vi "Convert API String Arguments to Data(variant).vi"(7 "Type":variant, 9 "error in (no error)":errorcluster, 10 "Strict Label Check?(T)":bool=TRUE, 11 "String":string) -> (1 "error":errorcluster, 3 "Data":variant)   [LabVIEW 2017, in "API String Arguments Support.lvlib"]
uses:
  API String Arguments Support.lvlib
  <vilib>/Utility/Data Type/Type Definitions/Data Type.ctl
  <vilib>/Utility/Data Type/Type Definitions/Tag Type.ctl
  <vilib>/Utility/Data Type/Type Definitions/Refnum Type.ctl
  <userlib>/_NEVSTOP/Communicable State Machine(CSM)/AdvanceAPI/CSM - Keywords.vi
  <vilib>/Utility/Data Type/NI_Data Type.lvlib
  <userlib>/_NEVSTOP/Communicable State Machine(CSM)/Communicable State Machine.lvlib
  <userlib>/_NEVSTOP/Communicable State Machine(CSM)/_Shared/CSM Shared.lvlib
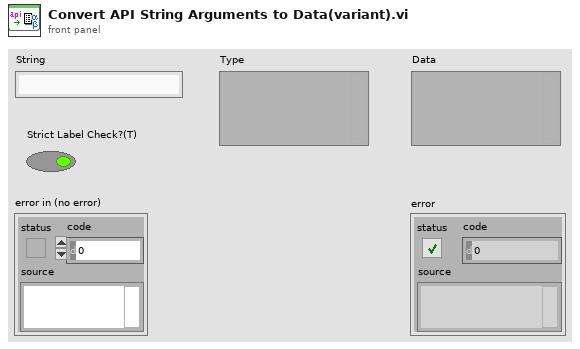
[diagram p1: front panel]
types:
  T1 = enum16{"0x2829 - ()", "0x5B5D - []", "0x7B7D - {}"}
  T2 = typedef "NI_Data Type.lvlib/Data Type.ctl" = enum8{"Invalid Type", "Void", "I8", "I16", "I32", "I64", "U8", "U16", "U32", "U64", "Single Float", "Double Float", "Extended Float", "Single Complex", "Double Complex", "Extended Complex", "Enum U8", "Enum U16", "Enum U32", "Enum U64", "Single Float With Unit", "Double Float With Unit", "Extended Float With Unit", "Single Complex with Unit", "Double Complex with Unit", "Extended Complex with Unit", "Boolean", "String", "Path", "Picture", "Tag", "Array", "Cluster", "Variant", "LV Variant", "Waveform", "Timestamp", "Digital Waveform", "Digital Data", "ExpressData", "Refnum", "External Data", "VI", "Poly VI", "LabVIEW Class Instance", "Fixed Point"}
  T3 = typedef "NI_Data Type.lvlib/Tag Type.ctl" = enum16{"kNoTagType", "\tkDSCTagType", "\tkOldDAQTagType", "\tkIVITagType", "\tkVISATagType", "\tkGenClassTagType", "\tkUnusedTagType1", "\tkFPTagType", "\tkMotionTagType", "\tkDAQmxTaskTagType", "\tkDAQmxChannelTagType", "\tkDAQmxScaleTagType", "\tkDAQmxDeviceTagType", "\tkDAQmxTerminalTagType", "\tkDAQmxPhysChanTagType", "\tkDAQmxTriggerTagType", "\tkDAQmxSwitchTagType", "\tkDAQmxSignalTagType", "\tkUnusedTagType2", "\tkCANTaskTagType", "\tkCANInterfaceTagType", "\tkCANChannelTagType", "\tkNumTagTypes"}
  T4 = typedef "NI_Data Type.lvlib/Refnum Type.ctl" = enum16{"NotARefnum", "UnknownRefnum", "Generic", "Datalog", "ByteStream", "Device", "Occurence", "TCPNetConnection", "Auto", "Menu", "Imaq", "Hardware", "DataSocket", "Visa", "IVI", "UDPNetConnection", "Notifier", "Queue", "Irda", "EventReg", "DotNet", "UserEvent", "Callback", "UNUSED_EMPTY_POSITION", "BlueToothNetConnection", "LVObjApp", "LVObjVI", "LVObjUnknown", "GenericClass", "UserDefinedRefnumTag", "DataValue", "RT FIFO", "TDMS File"}
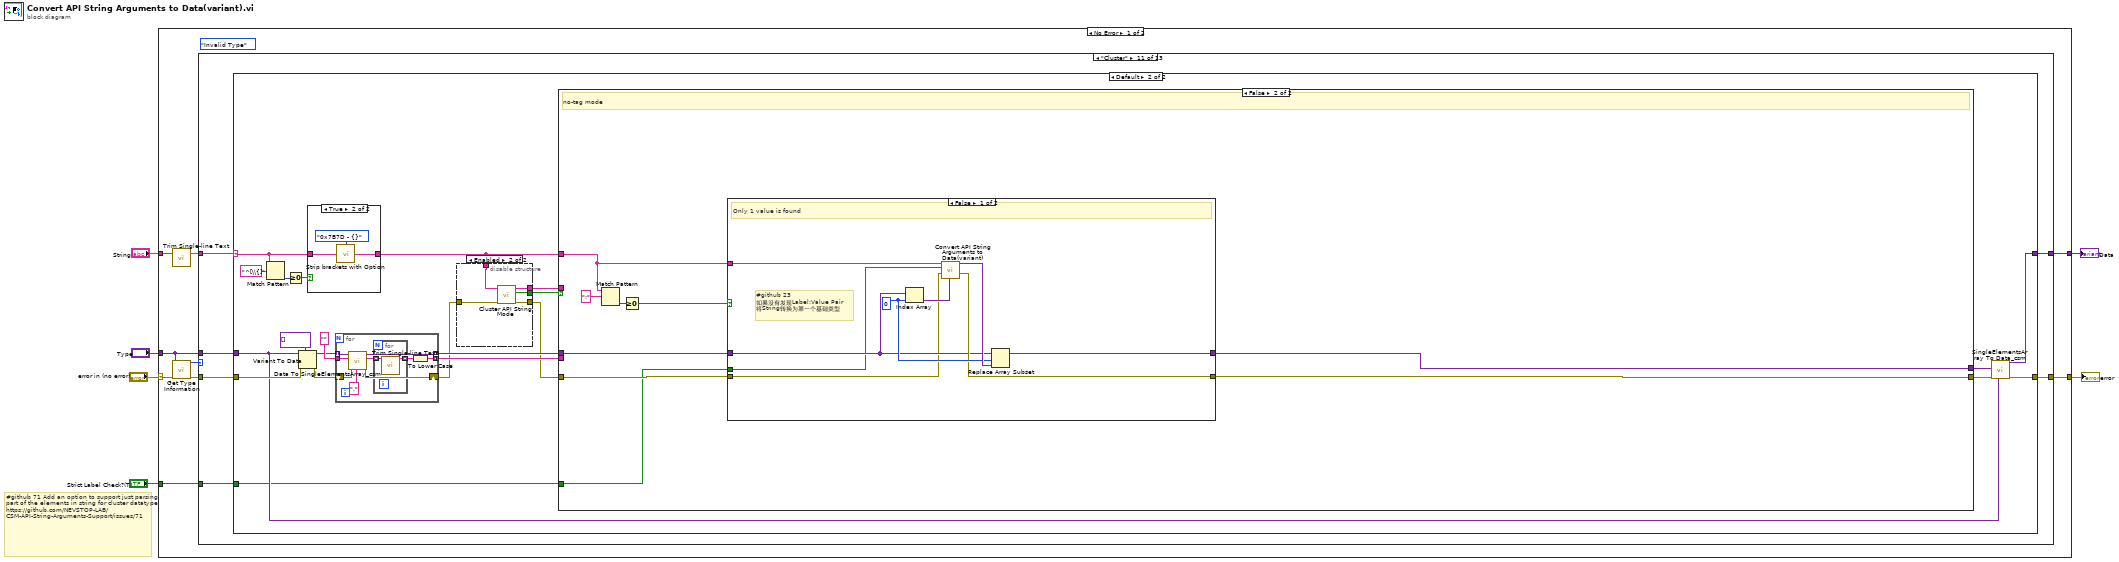
[diagram p0: block diagram]
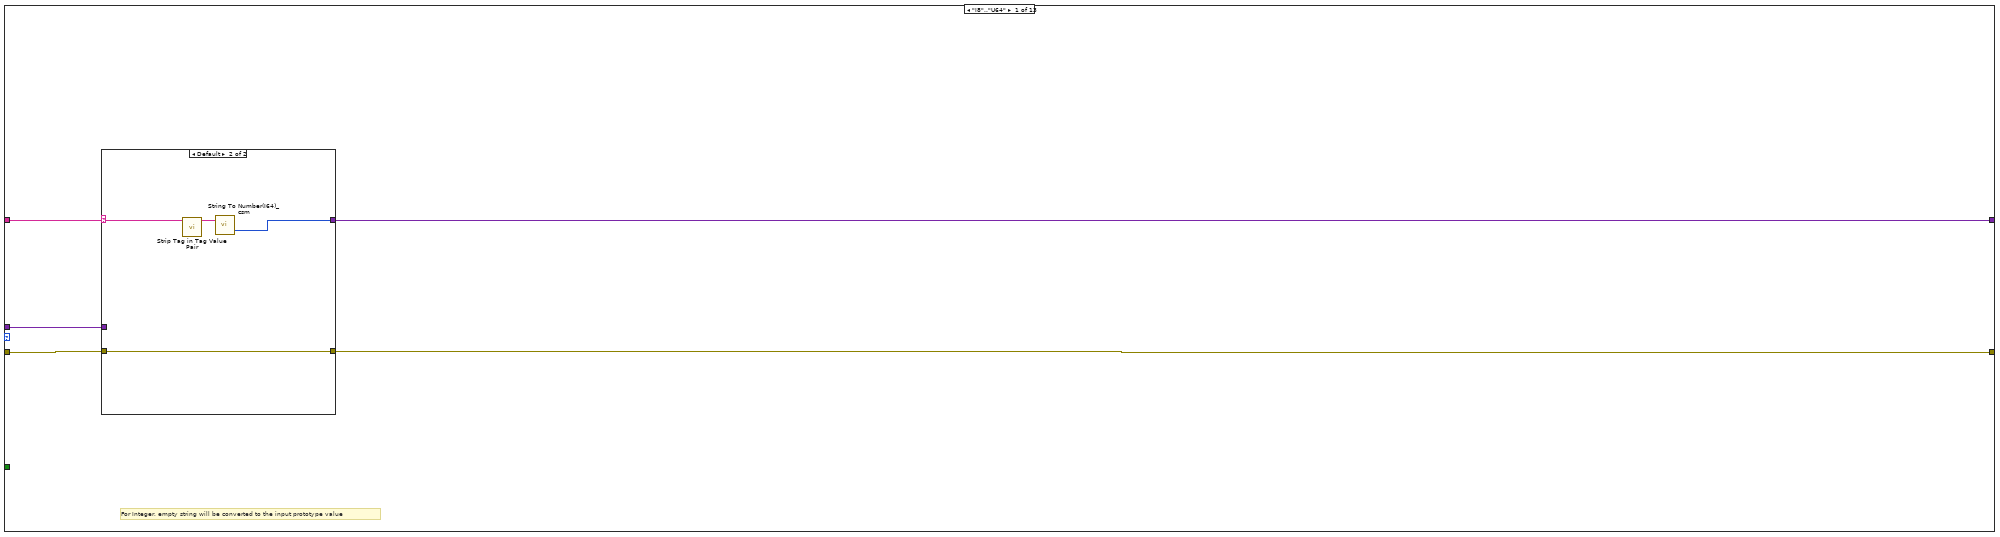
[diagram p2: hidden frame]
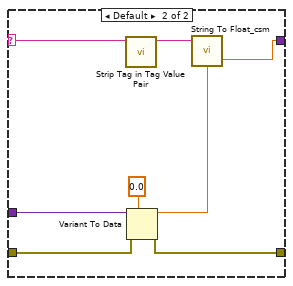
[diagram p5: hidden frame]
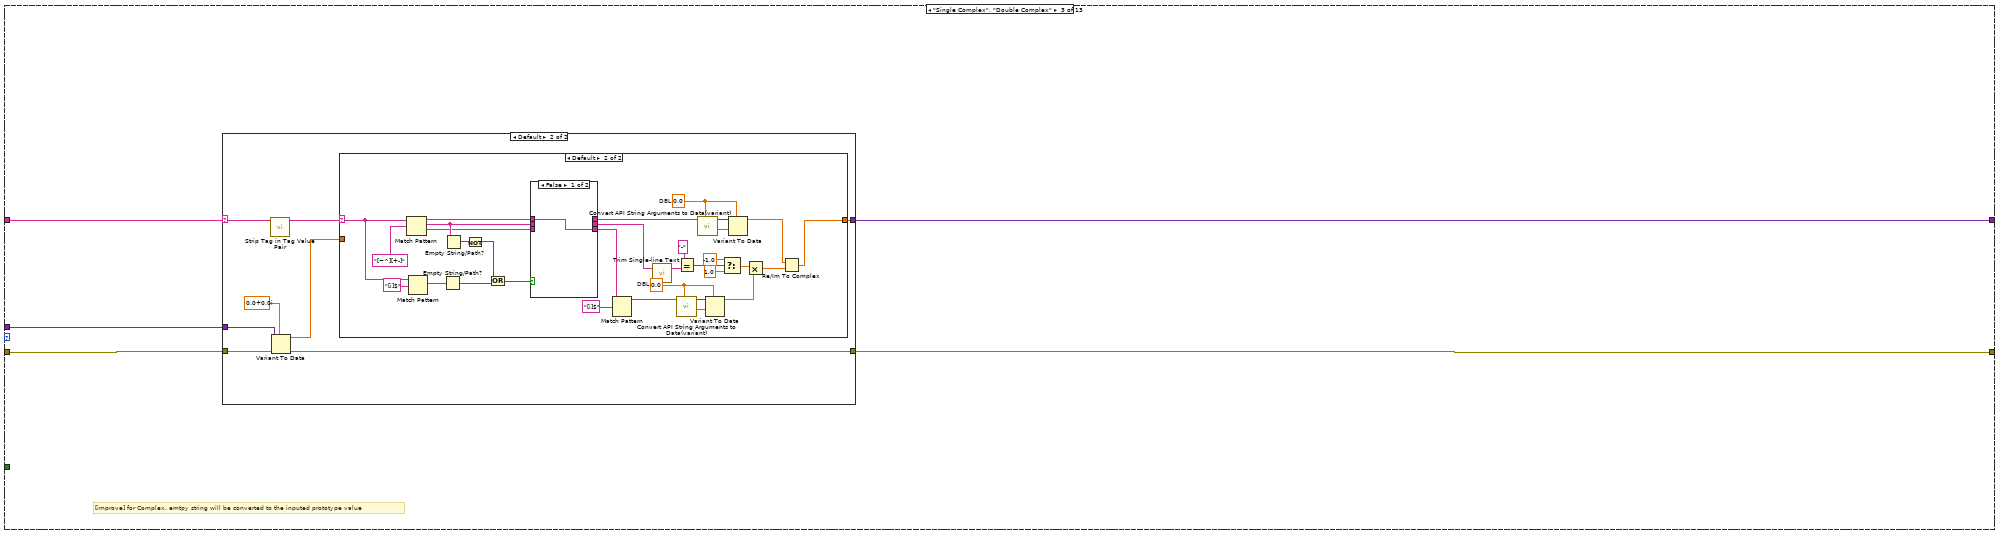
[diagram p6: hidden frame]
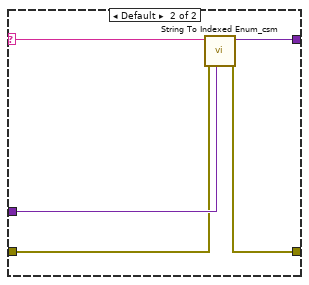
[diagram p11: hidden frame]
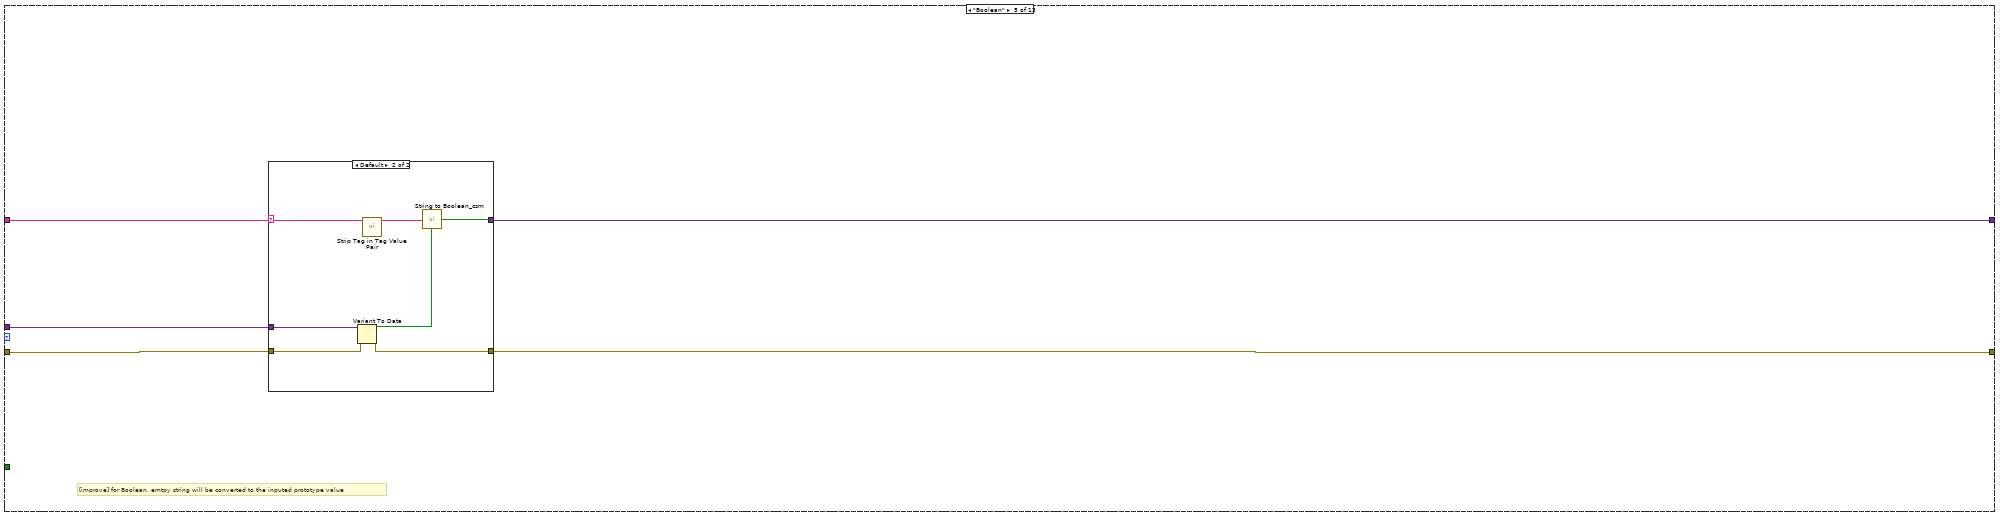
[diagram p12: hidden frame]
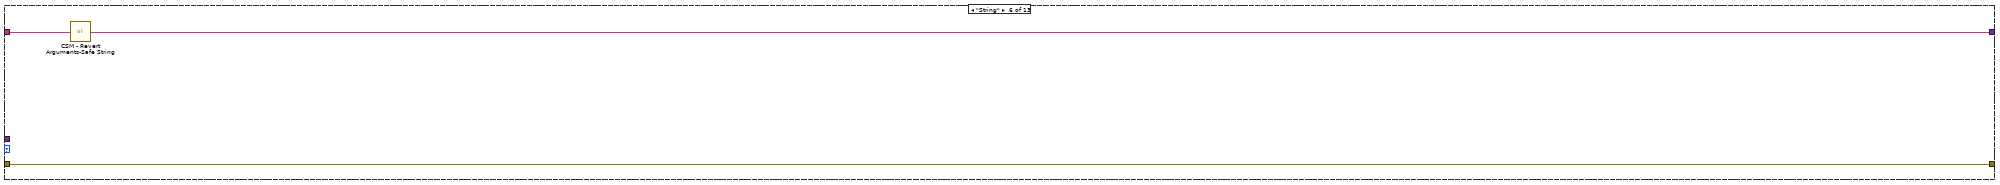
[diagram p14: hidden frame]
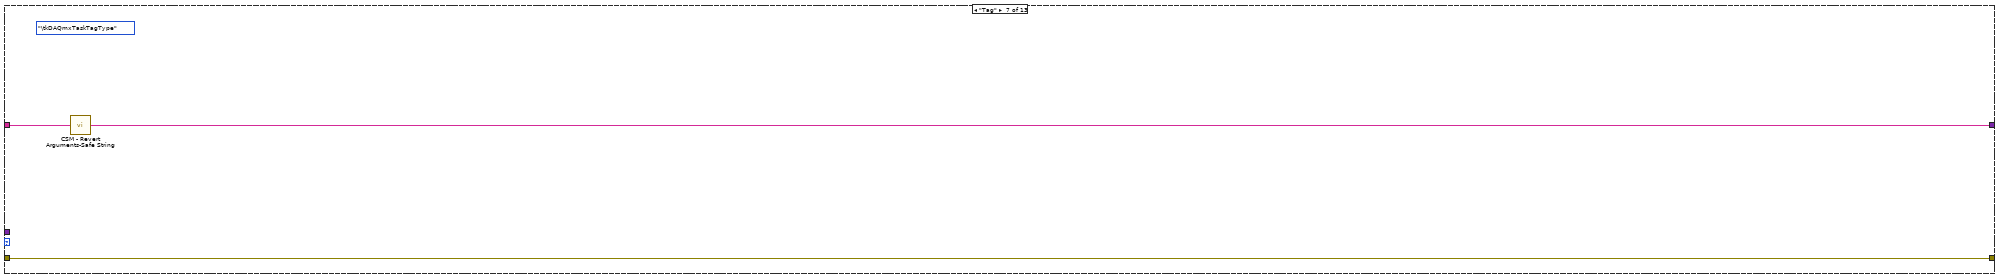
[diagram p15: hidden frame]
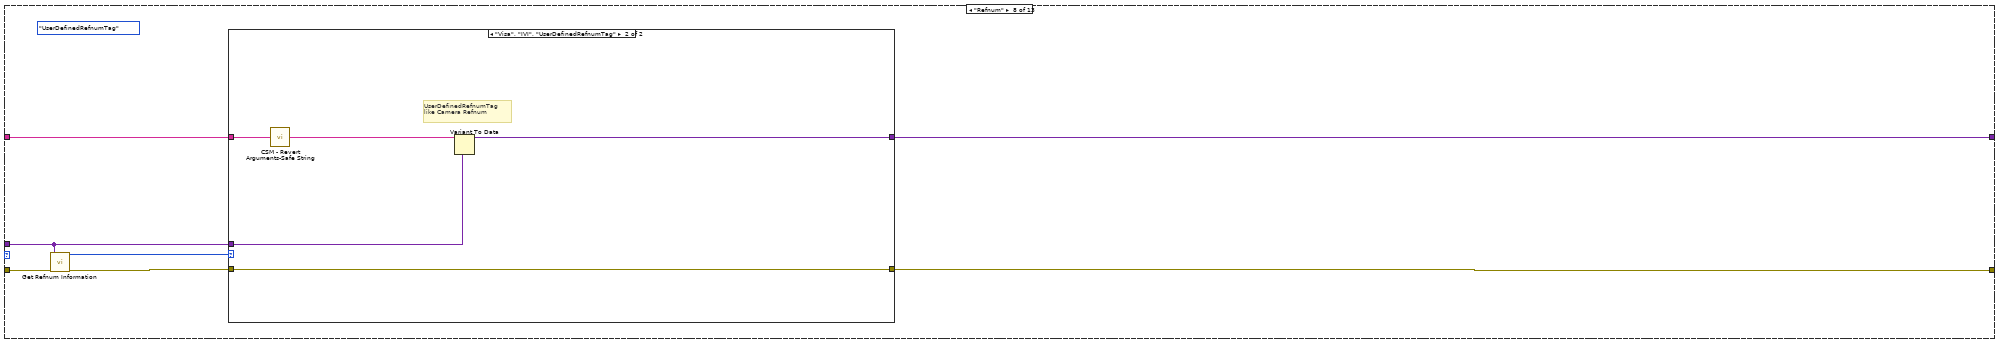
[diagram p16: hidden frame]
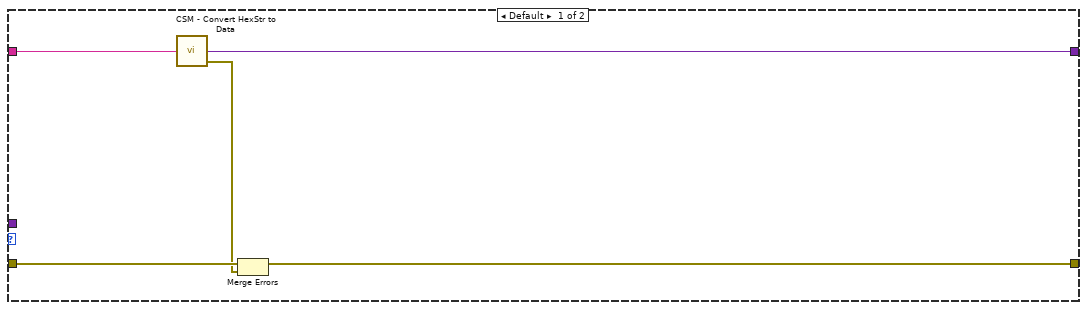
[diagram p17: hidden frame]
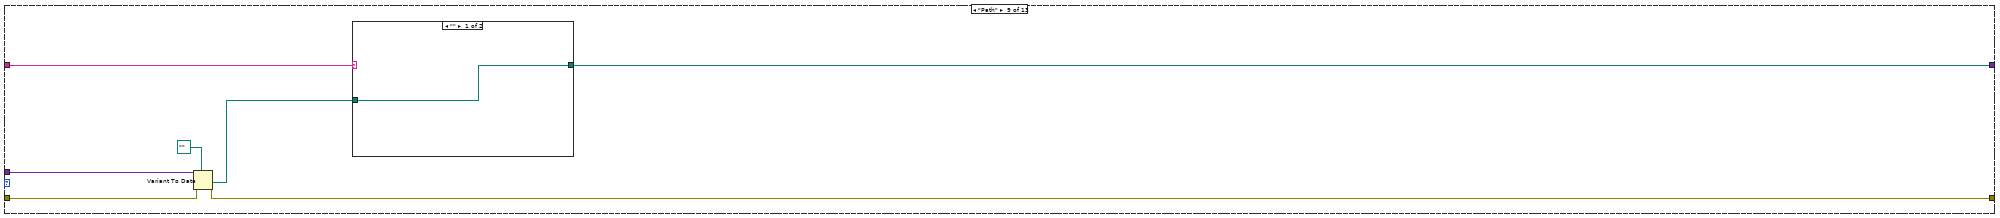
[diagram p18: hidden frame]
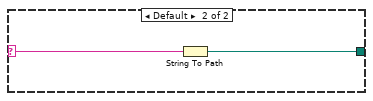
[diagram p19: hidden frame]
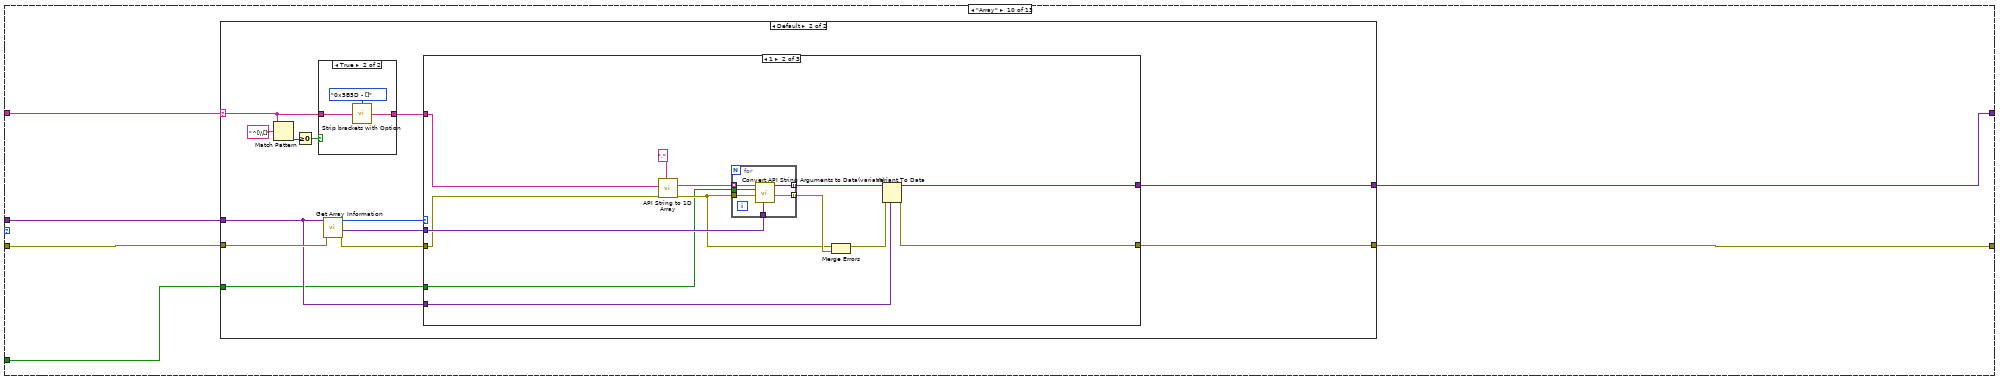
[diagram p20: hidden frame]
diagram:
  # "#github 71 Add an option to support just parsing part of the elements in string for cluster datatype\nhttps://github.com/NEVSTOP-LAB/CSM-API-String-Arguments-Support/issues/71"
  n1 = case shown="No Error" "error in (no error)" {
    selector: "error in (no error)" -> [w10 w619]
    tunnel: [w13 w619] -> w6
    tunnel: [w12 w618] -> w5
    tunnel: "Type" -> [w11 w618]
    tunnel: "String" -> [w9 _]
    tunnel: "Strict Label Check?(T)" -> [w7 _]
    frame No Error {
      (unwired) Data_Type."Invalid Type" ("type")
      n2 = call <userlib>:"Trim Single-line Text.vi"("single-line text"=w9) -> ("trimed text"=w8:string)  [unwired: 2 in]
      n3 = call <vilib>:"Get Type Information.vi"("error in (no error)"=w10, "Variant"=w11) -> ("error out"=w14:errorcluster, "Type"=w15:T2)  [unwired: 5 in, 3 out]
      n4 = case shown="\"Cluster\"" w15 {
        tunnel: w14 -> [w18 w31 w46 w96 w107 w122 w125 w132 w149 w158 w240 w570 w610]
        tunnel: [w17 w28 w44 w95 w106 w122 w125 w130 w146 w156 w243 w568 w607] -> w13
        tunnel: [w19 w29 w45 w94 w109 w120 w123 w127 w147 w157 w242 w569 w608] -> w12
        tunnel: w11 -> [w16 w27 w43 w97 w108 _ _ w129 w145 w155 w241 _ w606]
        tunnel: w8 -> [w20 w30 w42 w98 w110 w121 w124 w128 w148 w154 w239 w567 w609]
        tunnel: w7 -> [_ _ _ _ _ _ _ _ _ w153 w238 _ _]
        frame "I8".."U64" {
          # "For Integer, empty string will be converted to the input prototype value"
          n5 = case shown="Default" w20 {
            selector: w20 -> [_ w26]
            tunnel: [w22 w25] -> w19
            tunnel: w18 -> [w21 w24]
            tunnel: [w21 w24] -> w17
            tunnel: w16 -> [w22 _]
            frame "" {
            }
            frame Default {
              n6 = call "Strip Tag in Tag Value Pair.vi"("Tag:Value"=w26) -> ("Value"=w23:string)  [unwired: 10 in]
              n7 = call "String To Number(I64)_csm.vi"("String"=w23) -> ("Numeric"=w25:u64)  [unwired: 4 in]
            }
          }
        }
        frame "Single Float", "Double Float" {
          # "[improve] for SGL/DBL, emtpy string will be converted to the inputed prototype value"
          n8 = case shown="\"\"" w30 {
            selector: w30 -> [_ w40]
            tunnel: w31 -> [w33 w41]
            tunnel: [w32 w39] -> w29
            tunnel: [w33 w38] -> w28
            tunnel: w27 -> [w32 w37]
            frame "" {
            }
            frame Default {
              n9 = call "Strip Tag in Tag Value Pair.vi"("Tag:Value"=w40) -> ("Value"=w34:string)  [unwired: 10 in]
              n10 = Variant To Data(error in=w41, type=0.0 ("Default(0)"), Variant=w37) -> (data=w35:dbl, error out=w38:errorcluster)
              n11 = call "String To Float_csm.vi"("Default (0)"=w35, "String"=w34) -> ("Float"=w39:dbl)  [unwired: 2 in, 1 out]
            }
          }
        }
        frame "Single Complex", "Double Complex" {
          # "[improve] for Complex, emtpy string will be converted to the inputed prototype value"
          n12 = case shown="Default" w42 {
            selector: w42 -> [_ w50]
            tunnel: w46 -> [w48 w56]
            tunnel: [w47 w55] -> w45
            tunnel: [w48 w54] -> w44
            tunnel: w43 -> [w47 w53]
            frame "" {
            }
            frame Default {
              n13 = call "Strip Tag in Tag Value Pair.vi"("Tag:Value"=w50) -> ("Value"=w49:string)  [unwired: 10 in]
              n14 = Variant To Data(error in=w56, type=cdb 0.0+0.0i ("x + iy"), Variant=w53) -> (data=w51:cdb, error out=w54:errorcluster)
              n15 = case shown="Default" w49 {
                selector: w49 -> [_ w71]
                tunnel: [w57 w73] -> w55
                tunnel: w51 -> [w57 _]
                frame "" {
                }
                frame Default {
                  w82 = 0.0  # DBL
                  w85 = 0.0  # DBL
                  n16 = Match Pattern(string=w71, regular expression="[~^][+-]") -> (before substring=w66:string, match substring=w62:string, after substring=w61:string)  [unwired: 1 in, 1 out]
                  n17 = Match Pattern(string=w71, regular expression="[i]$") -> (match substring=w69:string)  [unwired: 1 in, 3 out]
                  n18 = Empty String/Path?(string/path=w69) -> (empty?=w63:bool)
                  n19 = Empty String/Path?(string/path=w62) -> (empty?=w68:bool)
                  n20 = Not(x=w68) -> (.not. x?=w64:bool)
                  n21 = Or(x=w64, y=w63) -> (x .or. y?=w67:bool)
                  n22 = case shown="False" w67 {
                    tunnel: w66 -> [w90 w93]
                    tunnel: [_ w93] -> w65
                    tunnel: w62 -> [_ w92]
                    tunnel: [_ w92] -> w58
                    tunnel: w61 -> [_ w91]
                    tunnel: [w90 w91] -> w60
                    frame False {
                    }
                    frame True {
                    }
                  }
                  n23 = Match Pattern(string=w60, regular expression="[i]$") -> (before substring=w72:string)  [unwired: 1 in, 3 out]
                  n24 = call <userlib>:"Trim Single-line Text.vi"("single-line text"=w58) -> ("trimed text"=w59:string)  [unwired: 2 in]
                  n25 = call "Convert API String Arguments to Data(variant).vi"("Type"=w82, "String"=w72) -> ("error"=w84:errorcluster, "Data"=w83:variant)  [unwired: 8 in]
                  n26 = Equal?(x="-", y=w59) -> (x = y?=w79:bool)
                  n27 = call "Convert API String Arguments to Data(variant).vi"("Type"=w85, "String"=w65) -> ("error"=w87:errorcluster, "Data"=w86:variant)  [unwired: 8 in]
                  n28 = Variant To Data(error in=w84, type=w82, Variant=w83) -> (data=w81:dbl)  [unwired: 1 out]
                  n29 = Select(t=-1.0, s=w79, f=1.0 ("t")) -> (s? t:f=w78:dbl)
                  n30 = Variant To Data(error in=w87, type=w85, Variant=w86) -> (data=w74:dbl)  [unwired: 1 out]
                  n31 = Multiply(x=w78, y=w81) -> (x*y=w75:dbl)
                  n32 = Re/Im To Complex(1:w75, 2:w74) -> (0:w73:cdb)
                }
              }
            }
          }
        }
        frame "Enum U8".."Enum U64" {
          n33 = case shown="\"\"" w98 {
            selector: w98 -> [_ w105]
            tunnel: w97 -> [w100 w104]
            tunnel: w96 -> [w99 w103]
            tunnel: [w99 w102] -> w95
            tunnel: [w100 w101] -> w94
            frame "" {
            }
            frame Default {
              n34 = call "String To Indexed Enum_csm.vi"("Variant"=w104, "error in (no error)"=w103, "String"=w105) -> ("error out"=w102:errorcluster, "Enum"=w101:variant)  [unwired: 7 in]
            }
          }
        }
        frame "Boolean" {
          # "[improve] for Boolean, emtpy string will be converted to the inputed prototype value"
          n35 = case shown="Default" w110 {
            selector: w110 -> [_ w119]
            tunnel: [w112 w118] -> w109
            tunnel: w108 -> [w112 w117]
            tunnel: w107 -> [w111 w115]
            tunnel: [w111 w114] -> w106
            frame "" {
            }
            frame Default {
              n36 = Variant To Data(error in=w115, Variant=w117) -> (data=w116:bool, error out=w114:errorcluster)  [unwired: 1 in]
              n37 = call "Strip Tag in Tag Value Pair.vi"("Tag:Value"=w119) -> ("Value"=w113:string)  [unwired: 10 in]
              n38 = call "String to Boolean_csm.vi"("Default (F)"=w116, "String"=w113) -> ("Boolean"=w118:bool)  [unwired: 2 in]
            }
          }
        }
        frame "String" {
          n39 = call <userlib>:"CSM - Revert Arguments-Safe String.vi"("Safe Argument String"=w121) -> ("Origin Argument String"=w120:string)  [unwired: 8 in]
        }
        frame "Tag" {
          (unwired) Tag_Type."\tkDAQmxTaskTagType" ("Tag Type")
          n40 = call <userlib>:"CSM - Revert Arguments-Safe String.vi"("Safe Argument String"=w124) -> ("Origin Argument String"=w123:string)  [unwired: 8 in]
        }
        frame "Refnum" {
          (unwired) Refnum_Type."UserDefinedRefnumTag" ("Reference Type")
          n41 = call <vilib>:"Get Refnum Information.vi"("error in (no error)"=w132, "Variant"=w129) -> ("error out"=w131:errorcluster, "Reference Type"=w126:T4)  [unwired: 6 in, 2 out]
          n42 = case shown="\"Visa\", \"IVI\", \"UserDefinedRefnumTag\"" w126 {
            tunnel: w131 -> [w137 w142]
            tunnel: [w135 w140] -> w127
            tunnel: [w134 w142] -> w130
            tunnel: w129 -> [_ w141]
            tunnel: w128 -> [w136 w139]
            frame Default {
              n43 = call <userlib>:"CSM - Convert HexStr to Data.vi"("HEX String"=w136) -> ("Variant"=w135:variant, "error out"=w133:errorcluster)  [unwired: 7 in]
              n44 = Merge Errors(w137, w133) -> (w134:errorcluster)
            }
            frame "Visa", "IVI", "UserDefinedRefnumTag" {
              # "UserDefinedRefnumTag\nlike Camera Refnum"
              n45 = call <userlib>:"CSM - Revert Arguments-Safe String.vi"("Safe Argument String"=w139) -> ("Origin Argument String"=w138:string)  [unwired: 8 in]
              n46 = Variant To Data(type=w141, Variant=w138) -> (data=w140:variant)  [unwired: 1 in, 1 out]
            }
          }
        }
        frame "Path" {
          n47 = Variant To Data(error in=w149, type=path "", Variant=w145) -> (data=w143:path, error out=w146:errorcluster)
          n48 = case shown="\"\"" w148 {
            selector: w148 -> [_ w152]
            tunnel: [w150 w151] -> w147
            tunnel: w143 -> [w150 _]
            frame "" {
            }
            frame Default {
              n49 = String To Path(string=w152) -> (path=w151:path)
            }
          }
        }
        frame "Array" {
          n50 = case shown="Default" w154 {
            selector: w154 -> [_ w163]
            tunnel: w158 -> [w160 w173]
            tunnel: [w159 w172] -> w157
            tunnel: [w160 w171] -> w156
            tunnel: w155 -> [w159 w167]
            tunnel: w153 -> [_ w161]
            frame "" {
            }
            frame Default {
              n51 = Match Pattern(string=w163, regular expression="^[\\[]") -> (offset past match=w166:i32)  [unwired: 1 in, 3 out]
              n52 = Greater Or Equal To 0?(x=w166) -> (x >= 0?=w165:bool)
              n53 = case shown="True" w165 {
                tunnel: [w234 w235] -> w162
                tunnel: w163 -> [w234 w237]
                frame False {
                }
                frame True {
                  n54 = call "Strip brackets with Option.vi"("TYPE"=T1."0x5B5D - []", "trimmed string in"=w237) -> ("trimmed string out"=w235:string)  [unwired: 2 in]
                }
              }
              n55 = call <vilib>:"Get Array Information.vi"("error in (no error)"=w173, "Variant"=w167) -> ("error out"=w170:errorcluster, "Array Element Data Type"=w169:variant, "Number of Dimensions"=w168:i32)  [unwired: 6 in, 1 out]
              n56 = case shown="1" w168 {
                tunnel: w162 -> [_ w177 w199]
                tunnel: [w175 w187 w207] -> w172
                tunnel: [errorcluster {"status"=TRUE, "code"=-1, "source"="DataType is not supported."} ("error out") w185 w205] -> w171
                tunnel: w170 -> [_ w181 w204]
                tunnel: w169 -> [_ w184 w200]
                tunnel: w167 -> [w175 w182 w203]
                tunnel: w161 -> [_ w176 w195]
                frame Default {
                }
                frame 1 {
                  n57 = call "API String to 1D Array.vi"("delimiter"="," ("delimiter (Tab)"), "error in (no error)"=w181, "trimmed string in"=w177) -> ("error out"=w180:errorcluster, "Array of Strings"=w178:string[])  [unwired: 7 in]
                  n58 = for {
                    tunnel: w178 -> [w191] mode=indexing
                    tunnel: [w193] -> w188 mode=indexing
                    tunnel: [w192] -> w183 mode=indexing
                    tunnel: w184 -> [w194]
                    tunnel: w180 -> [w190]
                    tunnel: w176 -> [w189]
                    n59 = call "Convert API String Arguments to Data(variant).vi"("Type"=w194, "error in (no error)"=w190, "Strict Label Check?(T)"=w189, "String"=w191) -> ("error"=w193:errorcluster, "Data"=w192:variant)  [unwired: 6 in]
                  }
                  n60 = Merge Errors(w180, w188) -> (w186:errorcluster)
                  n61 = Variant To Data(error in=w186, type=w182, Variant=w183) -> (data=w187:variant, error out=w185:errorcluster)
                }
                frame 2 {
                  n62 = call "API String to 1D Array.vi"("delimiter"=";" ("delimiter (Tab)"), "error in (no error)"=w204, "trimmed string in"=w199) -> ("error out"=w196:errorcluster, "Array of Strings"=w197:string[])  [unwired: 7 in]
                  n63 = for {
                    tunnel: [w217] -> w202 mode=indexing
                    tunnel: w200 -> [w216]
                    shift-right: [w218] -> w206
                    shift-left: w196 -> [w210]
                    tunnel: w197 -> [w212] mode=indexing
                    tunnel: w195 -> [w208]
                    n64 = call <userlib>:"Trim Single-line Text.vi"("single-line text"=w212) -> ("trimed text"=w211:string)  [unwired: 2 in]
                    n65 = call "API String to 1D Array.vi"("delimiter"="," ("delimiter (Tab)"), "error in (no error)"=w210, "trimmed string in"=w211) -> ("error out"=w209:errorcluster, "Array of Strings"=w214:string[])  [unwired: 7 in]
                    n66 = for {
                      tunnel: w214 -> [w222] mode=indexing
                      tunnel: [w224] -> w213 mode=indexing
                      tunnel: [w223] -> w217 mode=indexing
                      tunnel: w216 -> [w225]
                      tunnel: w209 -> [w220]
                      tunnel: w208 -> [w219]
                      n67 = call <userlib>:"Trim Single-line Text.vi"("single-line text"=w222) -> ("trimed text"=w221:string)  [unwired: 2 in]
                      n68 = call "Convert API String Arguments to Data(variant).vi"("Type"=w225, "error in (no error)"=w220, "Strict Label Check?(T)"=w219, "String"=w221) -> ("error"=w224:errorcluster, "Data"=w223:variant)  [unwired: 6 in]
                    }
                    n69 = Merge Errors(w209, w213) -> (w218:errorcluster)
                  }
                  n70 = for {
                    tunnel: w202 -> [w228] mode=indexing
                    tunnel: [w227] -> w201 mode=indexing
                    tunnel: w200 -> [w226]
                    n71 = for {
                      tunnel: w228 -> [w230] mode=indexing
                      tunnel: [w229] -> w227 mode=indexing
                      tunnel: w226 -> [w231]
                      n72 = Not Equal?(x=w230, y=variant ("Data")) -> (x != y?=w232:bool)
                      n73 = Select(t=w230, s=w232, f=w231) -> (s? t:f=w229:variant)
                    }
                  }
                  n74 = Variant To Data(error in=w206, type=w203, Variant=w201) -> (data=w207:variant, error out=w205:errorcluster)
                }
              }
            }
          }
        }
        frame "Cluster" {
          n75 = case shown="Default" w239 {
            selector: w239 -> [_ w257]
            tunnel: [w244 w266] -> w243
            tunnel: [w245 w264] -> w242
            tunnel: w241 -> [w245 w256]
            tunnel: w240 -> [w244 w259]
            tunnel: w238 -> [_ w250]
            frame "" {
            }
            frame Default {
              n76 = Match Pattern(string=w257, regular expression="^[\\{]") -> (offset past match=w262:i32)  [unwired: 1 in, 3 out]
              n77 = Greater Or Equal To 0?(x=w262) -> (x >= 0?=w261:bool)
              n78 = Variant To Data(error in=w259, type=variant[] [] ("Array"), Variant=w256) -> (data=w254:variant[], error out=w252:errorcluster)
              n79 = case shown="True" w261 {
                tunnel: [w563 w564] -> w258
                tunnel: w257 -> [w563 w566]
                frame False {
                }
                frame True {
                  n80 = call "Strip brackets with Option.vi"("TYPE"=T1."0x7B7D - {}", "trimmed string in"=w566) -> ("trimmed string out"=w564:string)  [unwired: 2 in]
                }
              }
              n81 = for {
                tunnel: [w558] -> w253 mode=concatenating
                tunnel: [w552] -> w251 mode=concatenating
                tunnel: "" ("parentUrl") -> [w555]
                tunnel: w254 -> [w554] mode=indexing
                shift-right: [w557] -> w247
                shift-left: w252 -> [w560]
                n82 = call "Data To SingleElementsArray_csm.vi"("Seperator(/)"=".", "error in (no error)"=w560, "parentUrl"=w555, "Cluster"=w554) -> ("error out"=w557:errorcluster, "Full NameList"=w556:string[], "DataElementArray"=w558:variant[])  [unwired: 5 in]
                n83 = for {
                  tunnel: w556 -> [w562] mode=indexing
                  tunnel: [w561] -> w553 mode=indexing
                  n84 = call <userlib>:"Trim Single-line Text.vi"("single-line text"=w562) -> ("trimed text"=w561:string)  [unwired: 2 in]
                }
                n85 = To Lower Case(string=w553) -> (all lower case string=w552:string[])
              }
              n86 = disable-structure shown="Enabled" {
                disable-tunnel: w258 -> [w545 w551]
                disable-tunnel: [w543 w550] -> w249
                disable-tunnel: [_ w549] -> w248
                disable-tunnel: w247 -> [w542 w548]
                disable-tunnel: [w542 w547] -> w246
                frame Disabled {
                  # "#github 23\n判断是否只有Label:Value Pair"
                  n87 = Match Pattern(string=w545, regular expression=":") -> (offset past match=w544:i32)  [unwired: 1 in, 3 out]
                  n88 = Greater Or Equal To 0?(x=w544) -> (x >= 0?=w543:bool)
                }
                frame Enabled {
                  n89 = call "Cluster API String Mode.vi"("error in (no error)"=w548, "cluster api string"=w551) -> ("error out"=w547:errorcluster, "TagValue Mode"=w550:bool, "Array of Strings"=w549:string[])  [unwired: 7 in]
                }
              }
              n90 = case shown="False" w249 {
                tunnel: [w275 w506] -> w267
                tunnel: [w274 w507] -> w265
                tunnel: w246 -> [w269 w501]
                tunnel: w258 -> [_ w503]
                tunnel: w253 -> [w273 w500]
                tunnel: w251 -> [w272 _]
                tunnel: w250 -> [w271 w499]
                tunnel: w248 -> [w268 _]
                frame True {
                  # "tag:value mode"
                  n91 = Empty Array?(array=w268) -> (empty?=w270:bool)
                  n92 = case shown="False" w270 {
                    tunnel: [w276 w279] -> w275
                    tunnel: [w277 w282] -> w274
                    tunnel: w273 -> [w276 w292]
                    tunnel: w272 -> [_ w291]
                    tunnel: w269 -> [w277 w290]
                    tunnel: w271 -> [_ w285]
                    tunnel: w268 -> [_ w278]
                    frame True {
                    }
                    frame False {
                      # "#github 25\nthrow error if data is not defined"
                      n93 = for {
                        tunnel: w278 -> [w496] mode=indexing
                        shift-right: [w497] -> w293
                        shift-left: variant -> [w498]
                        # "Clear error"
                        n94 = Match Pattern(string=w496, regular expression=":") -> (before substring=w493:string, after substring=w494:string)  [unwired: 1 in, 2 out]
                        n95 = call <userlib>:"Trim Single-line Text.vi"("single-line text"=w493) -> ("trimed text"=w491:string)  [unwired: 2 in]
                        n96 = call <userlib>:"Trim Single-line Text.vi"("single-line text"=w494) -> ("trimed text"=w492:string)  [unwired: 2 in]
                        n97 = To Lower Case(string=w491) -> (all lower case string=w490:string)
                        n98 = Set Variant Attribute(Variant=w498, name=w490, value=w492) -> (Variant out=w497:variant)  [unwired: 1 in, 2 out]
                      }
                      n99 = disable-structure shown="Enabled" {
                        disable-tunnel: w293 -> [w327 w441]
                        disable-tunnel: [w326 w440] -> w280
                        disable-tunnel: w292 -> [w325 w439]
                        disable-tunnel: w291 -> [w324 w438]
                        disable-tunnel: w290 -> [w323 w437]
                        disable-tunnel: [w322 w436] -> w289
                        disable-tunnel: w285 -> [w321 w435]
                        disable-tunnel: [w320 w433] -> w284
                        frame Enabled {
                          # "#github 55 make leaf element name is ok for data parsing \nhttps://github.com/NEVSTOP-LAB/CSM-API-String-Arguments-Support/issues/55 \n#github 76 [sub-cluster].[leaf-element name] is also OK now\nhttps://github.com/NEVSTOP-LAB/CSM-API-String-Arguments-Support/issues/76"
                          n100 = disable-structure shown="Enabled" {
                            disable-tunnel: w327 -> [w335 w395]
                            disable-tunnel: [w329 w394] -> w326
                            disable-tunnel: w325 -> [w334 w393]
                            disable-tunnel: w324 -> [w328 w392]
                            disable-tunnel: w323 -> [w333 w391]
                            disable-tunnel: [w332 w390] -> w322
                            disable-tunnel: w321 -> [w331 w389]
                            disable-tunnel: [w330 w387] -> w320
                            frame Enabled {
                              # "#github 86 use breadth-first traversal instead of depth-first traversal \nhttps://github.com/NEVSTOP-LAB/CSM-API-String-Arguments-Support/issues/86"
                              n101 = while {
                                shift-right: [w341] -> w332
                                shift-left: w335 -> [w348]
                                tunnel: w331 -> [w347]
                                shift-right: [w345] -> w329
                                shift-left: w334 -> [w346]
                                shift-right: [w340] -> _
                                shift-left: w328 -> [w344]
                                shift-right: [w343] -> w330
                                shift-left: w333 -> [w342]
                                stop <- w339 stop-if-true
                                n102 = for {
                                tunnel: w347 -> [w355]
                                shift-right: [w356] -> w341
                                shift-left: w348 -> [w358]
                                shift-right: [w354] -> w343
                                shift-left: w342 -> [w353]
                                tunnel: w346 -> [w351] mode=indexing
                                tunnel: [w349] -> w345 mode=indexing
                                tunnel: w344 -> [w352] mode=indexing
                                tunnel: [w350] -> w340 mode=indexing
                                n103 = case shown="Default" w352 {
                                selector: w352 -> [w359 w363]
                                tunnel: w358 -> [w361 w373]
                                tunnel: [_ w372] -> w357
                                tunnel: [w361 w370] -> w356
                                tunnel: w355 -> [_ w369]
                                tunnel: w351 -> [w360 w368]
                                tunnel: [w360 w367] -> w349
                                tunnel: [w359 w362] -> w350
                                frame "" {
                                }
                                frame Default {
                                n104 = Get Variant Attribute(Variant=w373, name=w363, default value (empty Variant)="" ("regular expression")) -> (duplicate Variant=w365:variant, found=w364:bool, value=w371:string)  [unwired: 1 in, 1 out]
                                n105 = case shown="False" w364 {
                                tunnel: [_ w386] -> w372
                                tunnel: w371 -> [_ w385]
                                tunnel: [w377 w384] -> w370
                                tunnel: w369 -> [_ w383]
                                tunnel: w368 -> [w378 w382]
                                tunnel: [w378 w381] -> w367
                                tunnel: w363 -> [_ w380]
                                tunnel: w365 -> [w377 w379]
                                tunnel: w363 -> [w376 _]
                                tunnel: [w374 _] -> w362
                                frame False {
                                n106 = Match Pattern(string=w376, regular expression="[.]" ("delimiter (Tab)")) -> (after substring=w374:string)  [unwired: 1 in, 3 out]
                                }
                                frame True {
                                n107 = call "Convert API String Arguments to Data(variant).vi"("Type"=w382, "Strict Label Check?(T)"=w383, "String"=w385) -> ("error"=w386:errorcluster, "Data"=w381:variant)  [unwired: 7 in]
                                n108 = Delete Variant Attribute(6:w380, 7:w379) -> (3:w384:variant)  [unwired: 1 in, 2 out]
                                }
                                }
                                }
                                }
                                n109 = Merge Errors(w353, w357) -> (w354:errorcluster)
                                }
                                n110 = Empty String/Path?(string/path=w341) -> (empty?=w338:bool)
                                n111 = Empty String/Path?(string/path=w340) -> (empty?=w337:bool[])
                                n112 = And Array Elements(Boolean array=w337) -> (logical AND=w336:bool)
                                n113 = Or(x=w338, y=w336) -> (x .or. y?=w339:bool)
                              }
                            }
                            frame Disabled {
                              n114 = for {
                                tunnel: w393 -> [w405] mode=indexing
                                tunnel: w391 -> [w397]
                                tunnel: w392 -> [w402] mode=indexing
                                tunnel: [w404] -> w394 mode=indexing
                                tunnel: [w403] -> w388 mode=indexing
                                shift-right: [w399] -> w390
                                shift-left: w395 -> [w406]
                                tunnel: w389 -> [w398]
                                n115 = while {
                                tunnel: [w410] -> w400
                                shift-right: [w420] -> w399
                                shift-left: w406 -> [w417]
                                tunnel: [w421] -> w401
                                shift-right: [w415] -> _
                                shift-left: w402 -> [w414]
                                shift-right: [w407] -> w396
                                shift-left: w397 -> [w408]
                                stop <- w413 stop-if-true
                                n116 = Match Pattern(string=w414, regular expression="[.]" ("delimiter (Tab)")) -> (after substring=w415:string, offset past match=w412:i32)  [unwired: 1 in, 2 out]
                                n117 = Get Variant Attribute(Variant=w417, name=w414, default value (empty Variant)="" ("regular expression"), error in=w408) -> (duplicate Variant=w418:variant, found=w410:bool, value=w421:string, error out=w407:errorcluster)
                                n118 = Less Than 0?(x=w412) -> (x < 0?=w411:bool)
                                n119 = Or(x=w410, y=w407) -> (x .or. y?=w409:bool)
                                n120 = case shown="True" w410 {
                                tunnel: [w422 w425] -> w420
                                tunnel: w418 -> [w422 w424]
                                tunnel: w414 -> [_ w423]
                                frame False {
                                }
                                frame True {
                                n121 = Delete Variant Attribute(6:w423, 7:w424) -> (3:w425:variant)  [unwired: 1 in, 2 out]
                                }
                                }
                                n122 = Or(x=w409, y=w411) -> (x .or. y?=w413:bool)
                                }
                                n123 = case shown="True" w400 {
                                tunnel: w405 -> [w427 w432]
                                tunnel: w401 -> [_ w429]
                                tunnel: [w427 w431] -> w404
                                tunnel: [w426 w430] -> w403
                                tunnel: w396 -> [w426 _]
                                tunnel: w398 -> [_ w428]
                                frame False {
                                }
                                frame True {
                                n124 = call "Convert API String Arguments to Data(variant).vi"("Type"=w432, "Strict Label Check?(T)"=w428, "String"=w429) -> ("error"=w430:errorcluster, "Data"=w431:variant)  [unwired: 7 in]
                                }
                                }
                              }
                              n125 = Merge Errors(w388) -> (w387:errorcluster)
                            }
                          }
                        }
                        frame Disabled {
                          n126 = for {
                            tunnel: w439 -> [w453] mode=indexing
                            tunnel: w437 -> [w444]
                            tunnel: w438 -> [w449] mode=indexing
                            tunnel: [w452] -> w440 mode=indexing
                            tunnel: [w451] -> w434 mode=indexing
                            shift-right: [w443] -> w436
                            shift-left: w441 -> [w455]
                            tunnel: w435 -> [w442]
                            # "#github 55 make leaf element name is ok for data parsing \nhttps://github.com/NEVSTOP-LAB/CSM-API-String-Arguments-Support/issues/55"
                            n127 = Get Variant Attribute(Variant=w455, name=w449, default value (empty Variant)="" ("regular expression")) -> (duplicate Variant=w450:variant, found=w448:bool, value=w447:string)  [unwired: 1 in, 1 out]
                            n128 = case shown="False" w448 {
                              tunnel: w450 -> [w466 w470]
                              tunnel: w449 -> [w465 w468]
                              tunnel: w447 -> [_ w472]
                              tunnel: [w459 w472] -> w446
                              tunnel: [w460 TRUE] -> w445
                              tunnel: [w456 w469] -> w443
                              frame False {
                                n129 = call <userlib>:"String to 1D Array_csm.vi"("delimiter (Tab)"=".", "string"=w465) -> ("Array of Strings"=w462:string[])  [unwired: 9 in]
                                n130 = Array Size(array=w462) -> (size(s)=w463:i32)
                                n131 = Decrement(x=w463) -> (x-1=w461:i32)
                                n132 = Index Array(array=w462, index=w461) -> (element=w458:string)
                                n133 = Get Variant Attribute(Variant=w466, name=w458, default value (empty Variant)="" ("regular expression")) -> (duplicate Variant=w457:variant, found=w460:bool, value=w459:string)  [unwired: 1 in, 1 out]
                                n134 = Delete Variant Attribute(6:w458, 7:w457) -> (3:w456:variant)  [unwired: 1 in, 2 out]
                              }
                              frame True {
                                n135 = Delete Variant Attribute(6:w468, 7:w470) -> (3:w469:variant)  [unwired: 1 in, 2 out]
                              }
                            }
                            n136 = case shown="True" w445 {
                              tunnel: w453 -> [w474 w479]
                              tunnel: w446 -> [_ w476]
                              tunnel: [w474 w478] -> w452
                              tunnel: [w473 w477] -> w451
                              tunnel: w444 -> [w473 _]
                              tunnel: w442 -> [_ w475]
                              frame False {
                              }
                              frame True {
                                n137 = call "Convert API String Arguments to Data(variant).vi"("Type"=w479, "Strict Label Check?(T)"=w475, "String"=w476) -> ("error"=w477:errorcluster, "Data"=w478:variant)  [unwired: 7 in]
                              }
                            }
                          }
                          n138 = Merge Errors(w434) -> (w433:errorcluster)
                        }
                      }
                      n139 = Get Variant Attribute(Variant=w289) -> (names=w281:string[])  [unwired: 3 in, 3 out]
                      n140 = Empty Array?(array=w281) -> (empty?=w287:bool)
                      n141 = Not(x=w287) -> (.not. x?=w286:bool)
                      n142 = And(x=w286, y=w285) -> (x .and. y?=w288:bool)
                      n143 = case shown="True" w288 {
                        tunnel: w284 -> [w480 w489]
                        tunnel: [w480 w484] -> w283
                        tunnel: w281 -> [_ w482]
                        frame False {
                        }
                        frame True {
                          n144 = call <userlib>:"1D Array to String_csm.vi"("delimiter (Tab)"=",", "Array of Strings"=w482) -> ("delimited string"=w483:string)  [unwired: 9 in]
                          n145 = Format Into String(format string="\"%s\" is not defined in Cluster prototype. ", w483) -> (resulting string=w486:string)  [unwired: 2 in, 1 out]
                          n146 = call <userlib>:"Build Error Cluster.vi"("String to Prepend to Source (\"\")"=w486, "Code"=-1 ("code")) -> ("error out"=w488:errorcluster)
                          n147 = Merge Errors(w489, w488) -> (w484:errorcluster)
                        }
                      }
                      n148 = case shown="Error" w283 {
                        selector: w283 -> [w296 w300]
                        tunnel: [w296 w299] -> w282
                        tunnel: w278 -> [_ w303]
                        tunnel: w280 -> [w295 w301]
                        tunnel: [w295 w302] -> w279
                        frame No Error {
                        }
                        frame Error {
                          # "Catch the finial opertunity to deal with some cases"
                          n149 = Array Size(array=w303) -> (size(s)=w304:i32)
                          n150 = Array Size(array=w301) -> (size(s)=w298:i32)
                          n151 = Equal?(x=w304, y=w298) -> (x = y?=w297:bool)
                          n152 = case shown="True" w297 {
                            tunnel: w303 -> [_ w313]
                            tunnel: [w306 w311] -> w302
                            tunnel: w301 -> [w306 w312]
                            tunnel: w300 -> [w305 w307]
                            tunnel: [w305 w308] -> w299
                            frame False {
                            }
                            frame True {
                              # "#github 84 \nhttps://github.com/NEVSTOP-LAB/CSM-API-String-Arguments-Support/issues/84"
                              n153 = for {
                                tunnel: w313 -> [w319] mode=indexing
                                tunnel: w312 -> [w318] mode=indexing
                                tunnel: [w317] -> w311 mode=indexing
                                tunnel: [w316] -> w310 mode=indexing
                                n154 = call "Convert API String Arguments to Data(variant).vi"("Type"=w318, "String"=w319) -> ("error"=w316:errorcluster, "Data"=w317:variant)  [unwired: 8 in]
                              }
                              n155 = Merge Errors(w310) -> (w309:errorcluster)
                              n156 = case shown="No Error" w309 {
                                selector: w309 -> [w314 _]
                                tunnel: [w314 w315] -> w308
                                tunnel: w307 -> [_ w315]
                                frame No Error {
                                }
                                frame Error {
                                }
                              }
                            }
                          }
                        }
                      }
                    }
                  }
                }
                frame False {
                  # "no-tag mode"
                  n157 = Match Pattern(string=w503, regular expression=";") -> (offset past match=w505:i32)  [unwired: 1 in, 3 out]
                  n158 = Greater Or Equal To 0?(x=w505) -> (x >= 0?=w502:bool)
                  n159 = case shown="False" w502 {
                    tunnel: w500 -> [w510 w527]
                    tunnel: w501 -> [w509 w518]
                    tunnel: [w513 w522] -> w507
                    tunnel: [w512 w523] -> w506
                    tunnel: w503 -> [w511 w521]
                    tunnel: w499 -> [w508 w517]
                    frame False {
                      w514 = 0 ("index")
                      # "#github 23\n如果没有发现Label:Value Pair\n将String转换为第一个基础类型"
                      # "Only 1 value is found"
                      n160 = Index Array(array=w510, index=w514) -> (element=w516:variant)
                      n161 = call "Convert API String Arguments to Data(variant).vi"("Type"=w516, "error in (no error)"=w509, "Strict Label Check?(T)"=w508, "String"=w511) -> ("error"=w513:errorcluster, "Data"=w515:variant)  [unwired: 6 in]
                      n162 = Replace Array Subset(array=w510, new element=w515, index=w514) -> (w512:variant[])
                    }
                    frame True {
                      # "Multiple values are found"
                      n163 = call "Cluster API String to 1D Array(Splite Nested Cluster).vi"("error in (no error)"=w518, "trimmed string in"=w521) -> ("error out"=w519:errorcluster, "Array of Strings"=w520:string[])  [unwired: 8 in]
                      n164 = Array Size(array=w520) -> (size(s)=w526:i32)
                      n165 = Array Size(array=w527) -> (size(s)=w525:i32)
                      n166 = Max & Min(x=w526, y=w525) -> (min(x,y)=w524:i32)  [unwired: 1 out]
                      n167 = for {
                        N: w524 -> [_]
                        shift-right: [w534] -> _
                        shift-left: w520 -> [w535]
                        shift-right: [w531] -> w523
                        shift-left: w527 -> [w533]
                        shift-right: [w530] -> w522
                        shift-left: w519 -> [w529]
                        tunnel: w517 -> [w528]
                        i -> [w532]
                        n168 = in-place {
                          in-place-border: [w538] -> w530
                          in-place-border: w529 -> [w537]
                          in-place-border: w528 -> [w536]
                          n169 = in-place-array #1(w535, w532) -> (w541:string)
                          n170 = in-place-array #2(w533, w532) -> (w540:variant)
                          n171 = call "Convert API String Arguments to Data(variant).vi"("Type"=w540, "error in (no error)"=w537, "Strict Label Check?(T)"=w536, "String"=w541) -> ("error"=w538:errorcluster, "Data"=w539:variant)  [unwired: 6 in]
                          n172 = in-place-array #1(w541) -> (w534:string[])  [unwired: 1 out]
                          n173 = in-place-array #2(w539) -> (w531:variant[])  [unwired: 1 out]
                        }
                      }
                    }
                  }
                }
              }
              n174 = call "SingleElementsArray To Data_csm.vi"("Pototype"=w256, "error in (no error)"=w265, "DataElementArray"=w267) -> ("error out"=w266:errorcluster, "Cluster"=w264:variant)  [unwired: 7 in]
            }
          }
        }
        frame "Timestamp" {
          n175 = case shown="Default" w567 {
            selector: w567 -> [_ w576]
            tunnel: w570 -> [w571 w579]
            tunnel: [w572 w578] -> w569
            tunnel: [w571 w577] -> w568
            frame "" {
              # "For Timestamp, empty string will be converted to current time."
              n176 = Get Date/Time In Seconds() -> (seconds since 1Jan1904=w572:timestamp)
            }
            frame Default {
              n177 = Match Pattern(string=w576, regular expression="^[0-9a-fA-F]$") -> (offset past match=w574:i32)  [unwired: 1 in, 3 out]
              n178 = Greater Or Equal To 0?(x=w574) -> (x >= 0?=w573:bool)
              n179 = case shown="False" w573 {
                tunnel: w579 -> [w585 w605]
                tunnel: [w586 w604] -> w578
                tunnel: [w584 w603] -> w577
                tunnel: w576 -> [w589 w601]
                frame False {
                  n180 = Match Pattern(string=w589, regular expression="(") -> (before substring=w583:string, after substring=w582:string)  [unwired: 1 in, 2 out]
                  n181 = Match Pattern(string=w582, regular expression=")") -> (before substring=w581:string)  [unwired: 1 in, 3 out]
                  n182 = call <userlib>:"Trim Single-line Text.vi"("single-line text"=w581) -> ("trimed text"=w580:string)  [unwired: 2 in]
                  n183 = case shown="\"\", \"UTC\"" w580 {
                    tunnel: w583 -> [w595 w600]
                    tunnel: w581 -> [w596 _]
                    tunnel: [w592 w599] -> w586
                    tunnel: w585 -> [w591 w597]
                    tunnel: [w590 w598] -> w584
                    frame Default {
                      w593 = timestamp(0 s since 1904-01-01) ("Time Stamp")
                      n184 = Scan From String(format string=w596, input string=w595, error in=w591, default 1=w593) -> (error out=w590:errorcluster, output 1=w594:timestamp)  [unwired: 1 in, 2 out]
                      n185 = Select(t=w593, s=w590, f=w594) -> (s? t:f=w592:timestamp)
                    }
                    frame "", "UTC" {
                      n186 = call "Text to Timestamp(RFC3339).vi"("error in (no error)"=w597, "Text Timestamp"=w600) -> ("error out"=w598:errorcluster, "Time Stamp"=w599:timestamp)  [unwired: 6 in, 2 out]
                    }
                  }
                }
                frame True {
                  n187 = call <userlib>:"CSM - Convert HexStr to Data.vi"("HEX String"=w601) -> ("Variant"=w604:variant, "error out"=w602:errorcluster)  [unwired: 7 in]
                  n188 = Merge Errors(w605, w602) -> (w603:errorcluster)
                }
              }
            }
          }
        }
        frame Default {
          n189 = case shown="Default" w609 {
            selector: w609 -> [w614 _]
            tunnel: w610 -> [w615 w617]
            tunnel: [w613 w616] -> w608
            tunnel: [w612 w617] -> w607
            tunnel: w606 -> [_ w616]
            frame Default {
              n190 = call <userlib>:"CSM - Convert HexStr to Data.vi"("HEX String"=w614) -> ("Variant"=w613:variant, "error out"=w611:errorcluster)  [unwired: 7 in]
              n191 = Merge Errors(w615, w611) -> (w612:errorcluster)
            }
            frame "" {
            }
          }
        }
      }
    }
    frame Error {
    }
  }
  "Data" <- w5
  "error" <- w6
